vi "Config.vi"() -> ()   [LabVIEW 2020]
uses:
  Database/Global1.vi
  Global_Variable/Global.vi
  Global_Variable/A131258.vi
  <vilib>/Utility/config.llb/NI_LVConfig.lvlib
panel:
  in  "系数":bool
  in  "产品型号":string(combo)
  in  "删除":bool
  in  "确定":bool
  in  "添加":bool
  in  "退出":bool
  in  "更新":bool
  in  "选项卡控件":enum32{"产品参数", "系统参数"}(tab)
  in  "启用第二段监控":bool
  in  "判定框范围":string[][](table)=[["°"], ["N"], ["°"], ["N"], ["°"], ["N"], ["°"], ["N"]]
  in  "结果判定参数":string[][](table)=[["N"], ["N"], ["N"], ["N"], ["N"], ["N"], ["N"], ["N"], ["N"]]
  in  "工位滤波":cluster{"启用滤波":bool, "滤波系数":dbl}
  in  "系统参数设置":string[][](table)=[[""], [""], [""], [""]]
  # "上转向轴组件压装"
types:
  T1 = enum8{"Enabled", "Disabled", "Disabled and Grayed Out"}
  T2 = typedef "NI_LVConfig.lvlib/Config Data RefNum.ctl" = refnum<k1>
  T3 = cluster{"用户编号":string, "用户名":string, "用户密码(密文)":string, "用户权限":string}
  T4 = cluster{"[0]":cluster{string, dbl, dbl}, "[1]":cluster{string, dbl, dbl}, "[2]":cluster{string, dbl, dbl}, "[3]":cluster{string, dbl, dbl}}
  T5 = cluster{"[0]":cluster{string, dbl, dbl}, "[1]":cluster{string, dbl, dbl}, "[2]":cluster{string, dbl, dbl}, "[3]":cluster{string, dbl, dbl}, "[4]":cluster{string, dbl, dbl}}
  T6 = cluster{"[0]":cluster{string, dbl, dbl}, "[1]":cluster{string, dbl, dbl}, "[2]":cluster{string, dbl, dbl}}
  T7 = cluster{"第一段判定框位移":cluster{"单位":string, "下限":dbl, "上限":dbl}, "第一段判定框压力":cluster{"单位":string, "下限":dbl, "上限":dbl}, "低二段判定框位移":cluster{"单位":string, "下限":dbl, "上限":dbl}, "第二段判定框压力":cluster{"单位":string, "下限":dbl, "上限":dbl}}
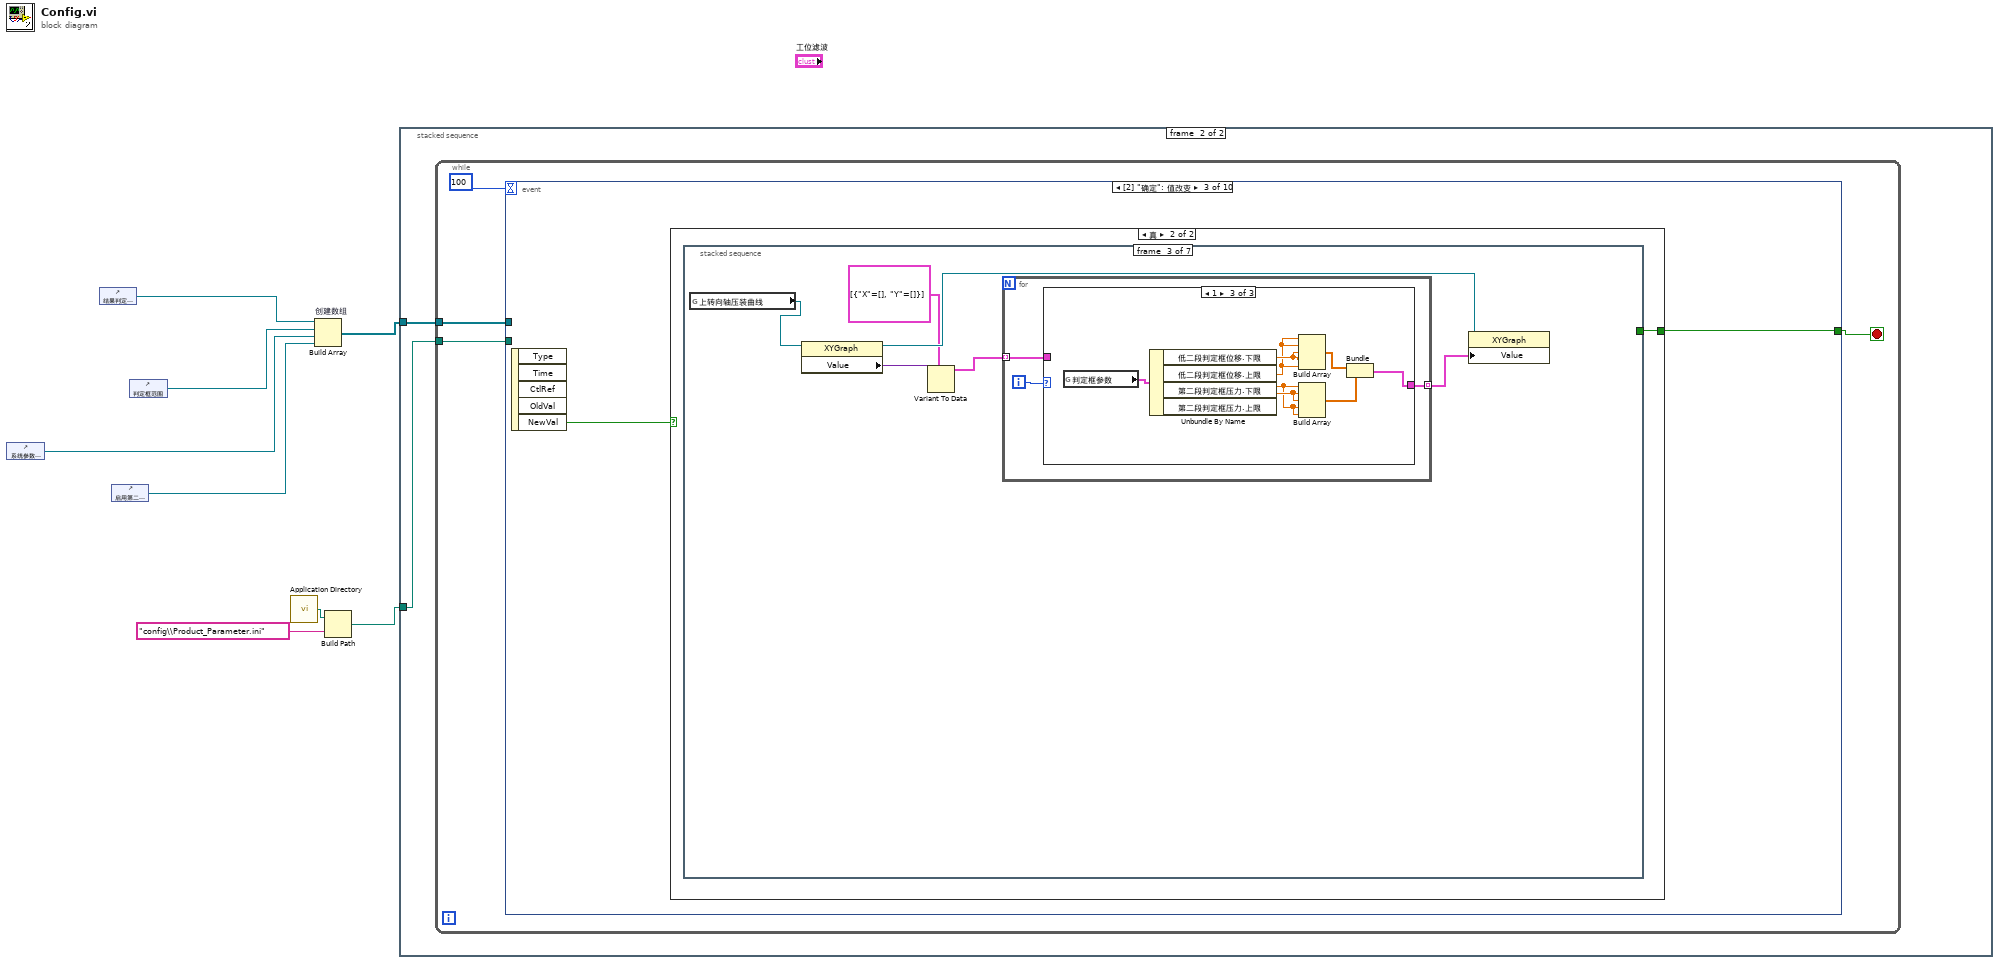
[diagram p0: block diagram]
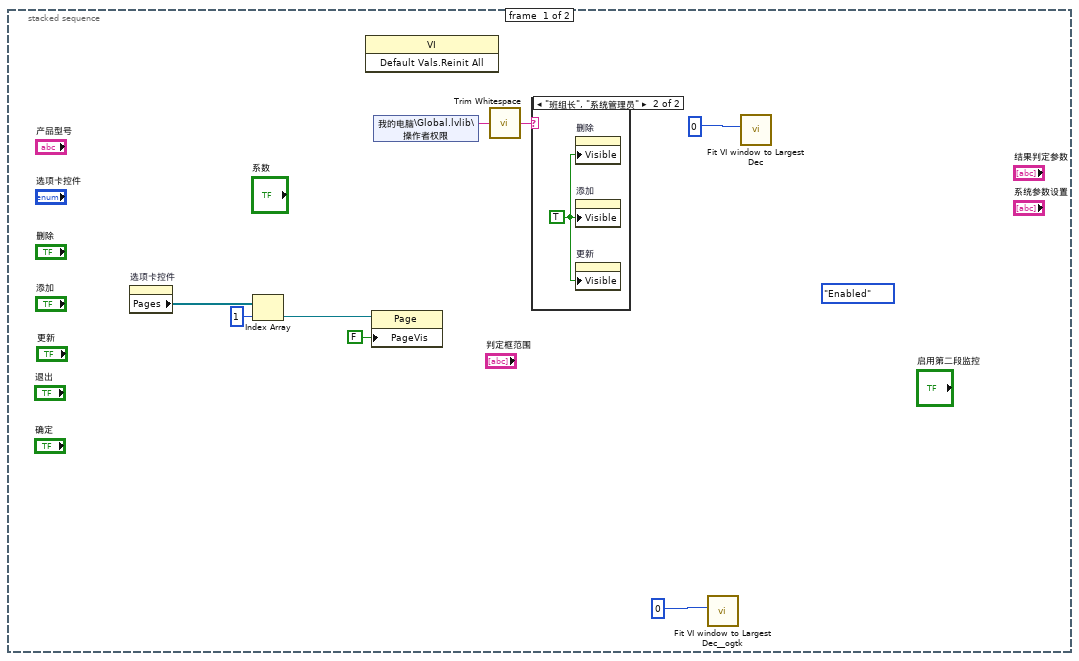
[diagram p2: hidden frame]
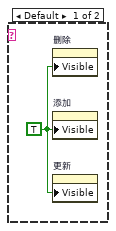
[diagram p3: hidden frame]
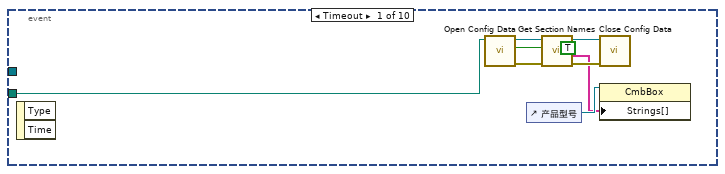
[diagram p4: hidden frame]
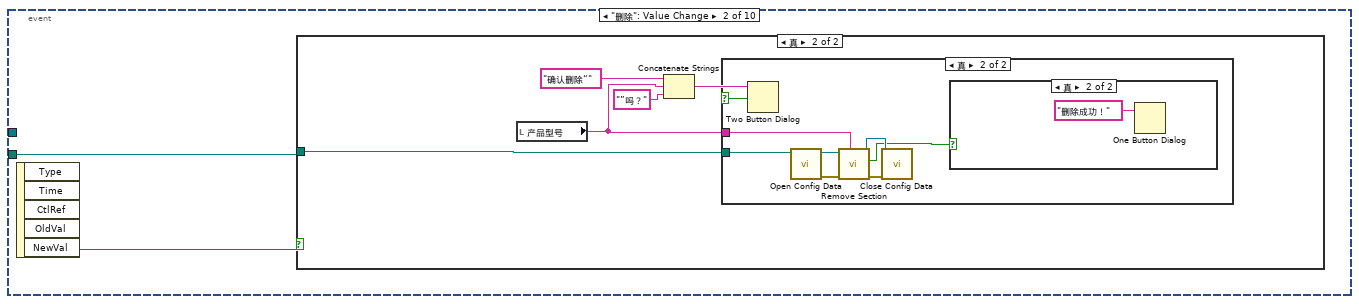
[diagram p5: hidden frame]
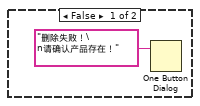
[diagram p8: hidden frame]
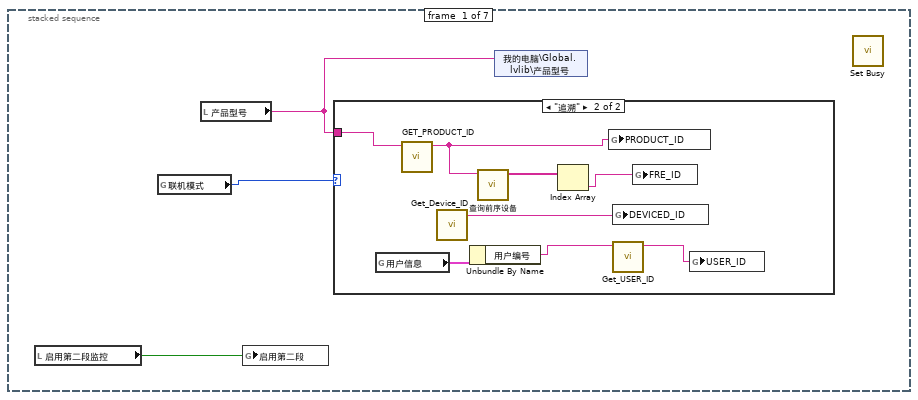
[diagram p10: hidden frame]
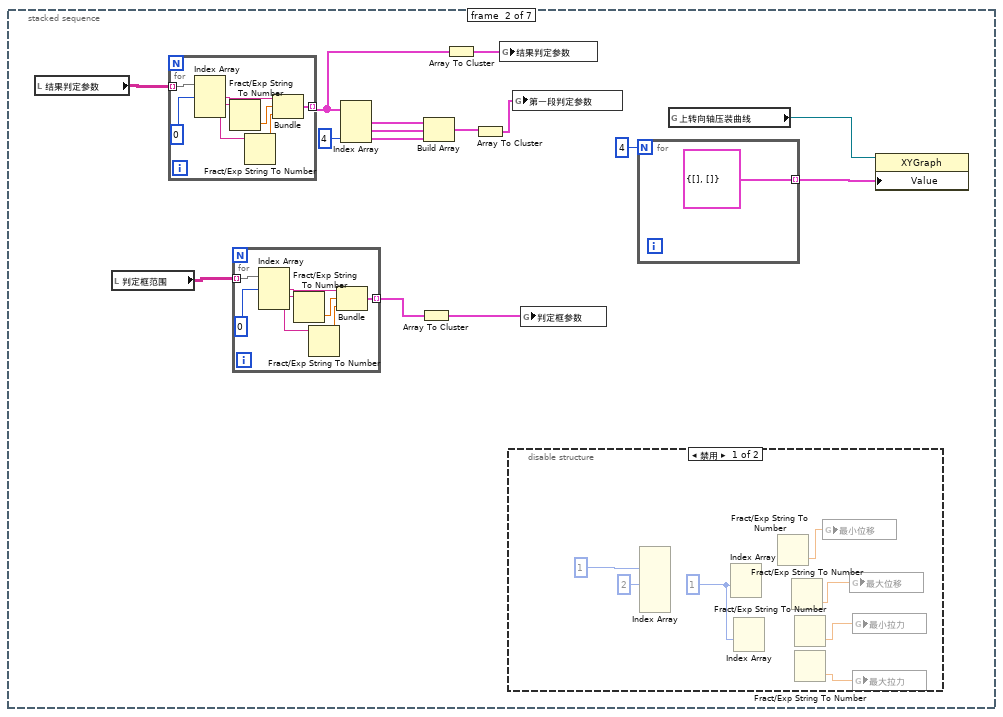
[diagram p12: hidden frame]
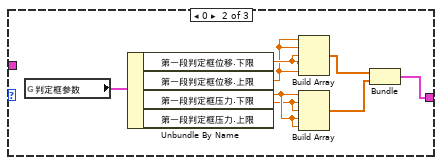
[diagram p15: hidden frame]
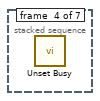
[diagram p16: hidden frame]
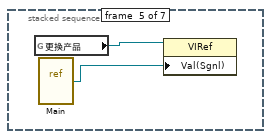
[diagram p17: hidden frame]
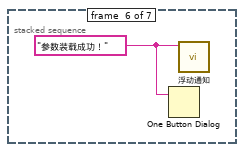
[diagram p18: hidden frame]
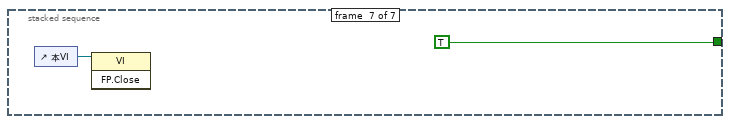
[diagram p19: hidden frame]
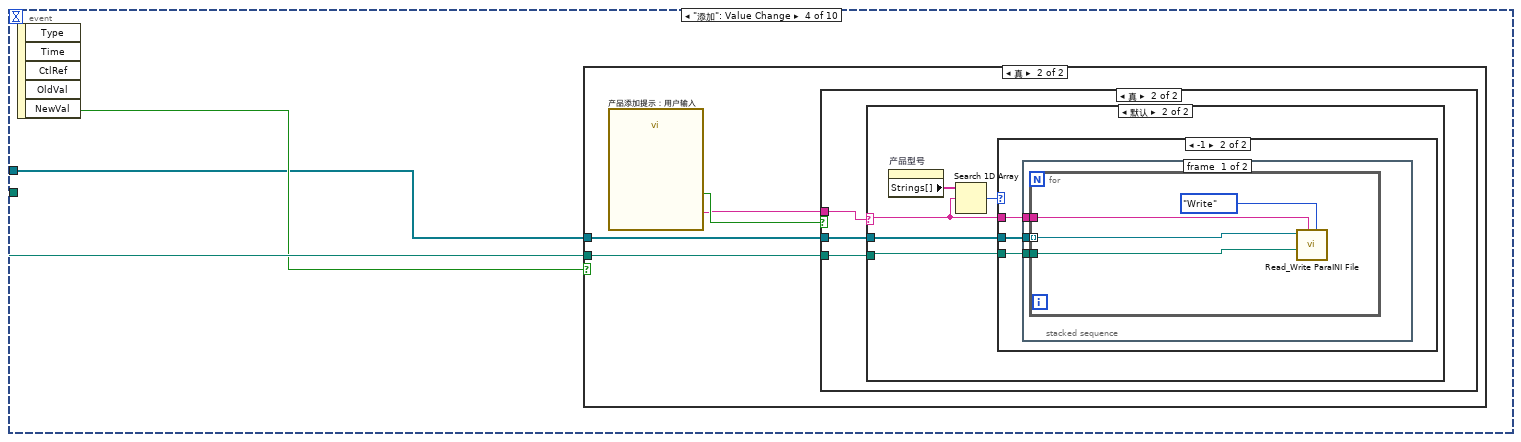
[diagram p20: hidden frame]
diagram:
  n1 = control-ref of="系统参数设置"() -> (w5:refnum<vi>)
  n2 = control-ref of="结果判定参数"() -> (w4:refnum<vi>)
  n3 = control-ref of="启用第二段监控"() -> (w1:refnum<vi>)
  n4 = control-ref of="判定框范围"() -> (w2:refnum<vi>)
  n5 = call <vilib>:"Application Directory.vi"() -> ("Application Directory"=w7:path)
  n6 = Build Array "创建数组"(w4, w2, w5, w1) -> (w8:refnum<vi>[])
  n7 = Build Path(base path=w7, name or relative path="config\\Product_Parameter.ini" ("名称或相对路径")) -> (appended path=w6:path)
  n8 = stacked-sequence {
    tunnel: w8 -> [_ w19]
    tunnel: w6 -> [_ w20]
    frame #0 {
      (unwired) T1."Enabled" ("禁用")
      n9 = property on="选项卡控件" class="TabCtl (严格)"() -> ("Pages"=w11:refnum<vi>[])  [unwired: 2 in, 2 out]
      n10 = Index Array(array=w11, index=1 ("索引")) -> (element=w12:refnum<vi>)
      n11 = invoke class="VI" method="Default Vals.Reinit All"() -> ()  [unwired: 3 in, 3 out]
      n12 = property class="Page"(reference=w12, "PageVis"=FALSE ("选项卡可见")) -> ()  [unwired: 1 in, 2 out]
      n13 = shared-variable "我的电脑\\Global.lvlib\\操作者权限"() -> (w16:string)  [unwired: 1 in, 1 out]
      n14 = call <vilib>:"Trim Whitespace.vi"("string"=w16) -> ("trimmed string"=w15:string)  [unwired: 1 in]
      n15 = case shown="\"班组长\", \"系统管理员\"" w15 {
        frame Default {
          w17 = TRUE ("可见")
          n16 = property on="删除" class="Bool (严格)"("Visible"=w17) -> ()  [unwired: 2 in, 2 out]
          n17 = property on="添加" class="Bool (严格)"("Visible"=w17) -> ()  [unwired: 2 in, 2 out]
          n18 = property on="更新" class="Bool (严格)"("Visible"=w17) -> ()  [unwired: 2 in, 2 out]
        }
        frame "班组长", "系统管理员" {
          w18 = TRUE ("可见")
          n19 = property on="删除" class="Bool (严格)"("Visible"=w18) -> ()  [unwired: 2 in, 2 out]
          n20 = property on="添加" class="Bool (严格)"("Visible"=w18) -> ()  [unwired: 2 in, 2 out]
          n21 = property on="更新" class="Bool (严格)"("Visible"=w18) -> ()  [unwired: 2 in, 2 out]
        }
      }
      n22 = call <userlib>:"Fit VI window to Largest Dec__ogtk.vi"("border spacing (2 px)"=0) -> ()  [unwired: 5 in, 2 out]
      n23 = call "Fit VI window to Largest Dec.vi"("border spacing (2 px)"=0) -> ()  [unwired: 5 in, 2 out]
    }
    frame #1 {
      n24 = while {
        tunnel: w20 -> [w24]
        tunnel: w19 -> [w21]
        stop <- w23 stop-if-true
        n25 = event shown="[2] \"确定\": 值改变" {
          selector: _ -> [_ _ _ _ _ _ _ _ _ _]
          dyn-events: _ -> [_ _ _ _ _ _ _ _ _ _]
          timeout: 100 -> [_ _ _ _ _ _ _ _ _ _]
          tunnel: w24 -> [w27 w34 _ w136 w164 _ w187 _ _ _]
          tunnel: [_ _ w50 _ _ TRUE _ _ _ TRUE] -> w23
          tunnel: w21 -> [_ _ _ w134 w162 _ w185 _ _ _]
          event Timeout {
            n26 = event-data() -> ()  [unwired: 1 in, 2 out]
            n27 = call <vilib>:"Open Config Data.vi"("create file if necessary (T)"=TRUE, "configuration file path"=w27) -> ("error out"=w29:errorcluster, "refnum"=w28:T2)  [unwired: 7 in, 1 out]
            n28 = control-ref of="产品型号"() -> (w26:refnum<vi>)
            n29 = call <vilib>:"Get Section Names.vi"("error in (no error)"=w29, "refnum"=w28) -> ("error out"=w31:errorcluster, "section names"=w25:string[], "refnum out"=w30:T2)  [unwired: 7 in]
            n30 = call <vilib>:"Close Config Data.vi"("error in (no error)"=w31, "refnum"=w30) -> ()  [unwired: 8 in, 2 out]
            n31 = property on="属性节点" class="CmbBox"(reference=w26, "Strings[]"=w25) -> ()  [unwired: 1 in, 2 out]
          }
          event "删除": Value Change {
            n32 = event-data() -> ("NewVal"=w33:bool)  [unwired: 1 in, 4 out]
            n33 = case shown="真" w33 {
              tunnel: w34 -> [_ w36]
              frame False {
              }
              frame True {
                n34 = local read "产品型号"() -> (w35:string)
                n35 = Concatenate Strings("确认删除“", w35, "”吗？") -> (w38:string)
                n36 = Two Button Dialog(message=w38) -> (T button?=w37:bool)  [unwired: 2 in]
                n37 = case shown="真" w37 {
                  tunnel: w36 -> [_ w42]
                  tunnel: w35 -> [_ w41]
                  frame False {
                  }
                  frame True {
                    n38 = call <vilib>:"Open Config Data.vi"("configuration file path"=w42) -> ("error out"=w44:errorcluster, "refnum"=w47:T2)  [unwired: 8 in, 1 out]
                    n39 = call <vilib>:"Remove Section.vi"("section"=w41, "error in (no error)"=w44, "refnum"=w47) -> ("error out"=w46:errorcluster, "section exists?"=w43:bool, "refnum out"=w45:T2)  [unwired: 6 in]
                    n40 = call <vilib>:"Close Config Data.vi"("error in (no error)"=w46, "refnum"=w45) -> ()  [unwired: 8 in, 2 out]
                    n41 = case shown="真" w43 {
                      frame False {
                        n42 = One Button Dialog(message="删除失败！\n请确认产品存在！" ("消息")) -> ()  [unwired: 1 in, 1 out]
                      }
                      frame True {
                        n43 = One Button Dialog(message="删除成功！" ("消息")) -> ()  [unwired: 1 in, 1 out]
                      }
                    }
                  }
                }
              }
            }
          }
          event "确定": Value Change {
            n44 = event-data() -> ("NewVal"=w51:bool)  [unwired: 1 in, 4 out]
            n45 = case shown="真" w51 {
              tunnel: [_ w52] -> w50
              frame False {
              }
              frame True {
                n46 = stacked-sequence {
                  tunnel: [_ _ _ _ _ _ TRUE] -> w52
                  frame #0 {
                    n47 = local read "启用第二段监控"() -> (w53:bool)
                    n48 = global read "Global1.vi" "联机模式"() -> (w55:enum16{"单机", "追溯"})
                    n49 = local read "产品型号"() -> (w54:string)
                    n50 = global write "Global.vi" "启用第二段"(w53) -> ()
                    n51 = case shown="\"追溯\"" w55 {
                      tunnel: w54 -> [_ w63]
                      frame "单机", Default {
                      }
                      frame "追溯" {
                        n52 = global read "Global1.vi" "用户信息"() -> (w61:T3)
                        n53 = call "GET_PRODUCT_ID.vi"("PRODFUCT_NAME"=w63) -> ("PRODUCT_ID"=w59:string)  [unwired: 10 in]
                        n54 = call "Get_Device_ID.vi"() -> ("Device_ID"=w57:string)  [unwired: 10 in, 1 out]
                        n55 = Unbundle By Name(w61) -> ("用户编号"=w60:string)
                        n56 = call "查询前序设备.vi"("PRODUCT_ID"=w59) -> ("前序工位"=w62:string[])  [unwired: 10 in]
                        n57 = Index Array(array=w62) -> (element=w58:string)  [unwired: 1 in]
                        n58 = global write "Global.vi" "PRODUCT_ID"(w59) -> ()
                        n59 = global write "Global.vi" "DEVICED_ID"(w57) -> ()
                        n60 = call "Get_USER_ID.vi"("USER_EMPLOYEE_ID"=w60) -> ("USER_ID"=w56:string)  [unwired: 9 in, 1 out]
                        n61 = global write "Global.vi" "FRE_ID"(w58) -> ()
                        n62 = global write "Global.vi" "USER_ID"(w56) -> ()
                      }
                    }
                    n63 = shared-variable "我的电脑\\Global.lvlib\\产品型号"(w54) -> ()  [unwired: 1 in, 1 out]
                    n64 = call <vilib>:"Set Busy.vi"() -> ()  [unwired: 10 in, 2 out]
                  }
                  frame #1 {
                    n65 = local read "结果判定参数"() -> (w78:string[][])
                    n66 = local read "判定框范围"() -> (w77:string[][])
                    n67 = for {
                      tunnel: w78 -> [w98] mode=indexing
                      tunnel: [w100] -> w68 mode=indexing
                      n68 = Index Array(array=w98, index #1=0) -> (element #1=w99:string, element #2=w97:string, element #3=w96:string)  [unwired: 2 in]
                      n69 = Fract/Exp String To Number(string=w97) -> (number=w102:dbl)  [unwired: 3 in, 1 out]
                      n70 = Fract/Exp String To Number(string=w96) -> (number=w101:dbl)  [unwired: 3 in, 1 out]
                      n71 = Bundle(w99, w102, w101) -> (w100:cluster{string, dbl, dbl})  [unwired: 1 in]
                    }
                    n72 = for {
                      tunnel: w77 -> [w90] mode=indexing
                      tunnel: [w92] -> w76 mode=indexing
                      n73 = Index Array(array=w90, index #1=0) -> (element #1=w91:string, element #2=w89:string, element #3=w88:string)  [unwired: 2 in]
                      n74 = Fract/Exp String To Number(string=w89) -> (number=w94:dbl)  [unwired: 3 in, 1 out]
                      n75 = Fract/Exp String To Number(string=w88) -> (number=w93:dbl)  [unwired: 3 in, 1 out]
                      n76 = Bundle(w91, w94, w93) -> (w92:cluster{string, dbl, dbl})  [unwired: 1 in]
                    }
                    n77 = Index Array(array=w68, index #3=4 ("索引")) -> (element #1=w71:cluster{string, dbl, dbl}, element #2=w70:cluster{string, dbl, dbl}, element #3=w69:cluster{string, dbl, dbl})  [unwired: 2 in]
                    n78 = Array To Cluster(array=w76) -> (cluster=w64:T4)
                    n79 = Build Array(w71, w70, w69) -> (w66:cluster{string, dbl, dbl}[])
                    n80 = Array To Cluster(array=w68) -> (cluster=w67:T5)
                    n81 = Array To Cluster(array=w66) -> (cluster=w65:T6)
                    n82 = global write "Global.vi" "结果判定参数"(w67) -> ()
                    n83 = disable-structure shown="禁用" {
                      frame Disabled {
                        w80 = 1 ("索引")
                        n84 = Index Array(index (row) #1=1 ("索引 (行)"), index (row) #2=2 ("索引 (行)")) -> ()  [unwired: 5 in, 3 out]
                        n85 = Index Array(index #1=w80) -> ()  [unwired: 2 in, 2 out]
                        n86 = Index Array(index #1=w80) -> ()  [unwired: 2 in, 2 out]
                        n87 = Fract/Exp String To Number() -> (number=w85:dbl)  [unwired: 4 in, 1 out]
                        n88 = Fract/Exp String To Number() -> (number=w84:dbl)  [unwired: 4 in, 1 out]
                        n89 = Fract/Exp String To Number() -> (number=w83:dbl)  [unwired: 4 in, 1 out]
                        n90 = Fract/Exp String To Number() -> (number=w82:dbl)  [unwired: 4 in, 1 out]
                        n91 = global write "判定参数.vi" "最小位移"(w85) -> ()
                        n92 = global write "判定参数.vi" "最大位移"(w84) -> ()
                        n93 = global write "判定参数.vi" "最小拉力"(w83) -> ()
                        n94 = global write "判定参数.vi" "最大拉力"(w82) -> ()
                      }
                      frame Enabled {
                      }
                    }
                    n95 = global write "Global.vi" "第一段判定参数"(w65) -> ()
                    n96 = global write "Global.vi" "判定框参数"(w64) -> ()
                    n97 = for {
                      N: 4 -> [_]
                      tunnel: [cluster{dbl[], dbl[]} {[], []}] -> w74 mode=indexing
                    }
                    n98 = global read "A131258.vi" "上转向轴压装曲线"() -> (w73:refnum<vi>)
                    n99 = property class="XYGraph"(reference=w73, "Value"=w74) -> ()  [unwired: 1 in, 2 out]
                  }
                  frame #2 {
                    n100 = global read "A131258.vi" "上转向轴压装曲线"() -> (w103:refnum<vi>)
                    n101 = property class="XYGraph"(reference=w103) -> (reference out=w108:refnum<vi>, "Value"=w106:variant)  [unwired: 1 in, 1 out]
                    n102 = Variant To Data(type=cluster{"X":dbl[], "Y":dbl[]}[] [{"X"=[], "Y"=[]}], Variant=w106) -> (data=w105:cluster{"X":dbl[], "Y":dbl[]}[])  [unwired: 1 in, 1 out]
                    n103 = for {
                      tunnel: [w110] -> w107 mode=indexing
                      tunnel: w105 -> [w109] mode=indexing
                      i -> [w111]
                      n104 = case shown="1" w111 {
                        tunnel: [w112 w113 w122] -> w110
                        tunnel: w109 -> [w112 _ _]
                        frame Default {
                        }
                        frame 0 {
                          n105 = global read "Global.vi" "判定框参数"() -> (w114:T7)
                          n106 = Unbundle By Name(w114) -> ("第一段判定框位移.下限"=w118:dbl, "第一段判定框位移.上限"=w117:dbl, "第一段判定框压力.下限"=w116:dbl, "第一段判定框压力.上限"=w115:dbl)
                          n107 = Build Array(w117, w117, w118, w118, w117) -> (w120:dbl[])
                          n108 = Build Array(w116, w115, w115, w116, w116) -> (w119:dbl[])
                          n109 = Bundle(w120, w119) -> (w113:cluster{dbl[], dbl[]})  [unwired: 1 in]
                        }
                        frame 1 {
                          n110 = global read "Global.vi" "判定框参数"() -> (w128:T7)
                          n111 = Unbundle By Name(w128) -> ("低二段判定框位移.下限"=w125:dbl, "低二段判定框位移.上限"=w121:dbl, "第二段判定框压力.下限"=w126:dbl, "第二段判定框压力.上限"=w127:dbl)
                          n112 = Build Array(w121, w121, w125, w125, w121) -> (w123:dbl[])
                          n113 = Build Array(w126, w127, w127, w126, w126) -> (w124:dbl[])
                          n114 = Bundle(w123, w124) -> (w122:cluster{dbl[], dbl[]})  [unwired: 1 in]
                        }
                      }
                    }
                    n115 = property class="XYGraph"(reference=w108, "Value"=w107) -> ()  [unwired: 1 in, 2 out]
                  }
                  frame #3 {
                    n116 = call <vilib>:"Unset Busy.vi"() -> ()  [unwired: 11 in, 1 out]
                  }
                  frame #4 {
                    n117 = global read "Global.vi" "更换产品"() -> (w130:refnum<vi>)
                    n118 = vi-ref "Main.vi"() -> (w129:refnum<vi>)
                    n119 = property class="VIRef"(reference=w130, "Val(Sgnl)"=w129) -> ()  [unwired: 1 in, 2 out]
                  }
                  frame #5 {
                    w131 = "参数装载成功！" ("消息")
                    n120 = One Button Dialog(message=w131) -> ()  [unwired: 1 in, 1 out]
                    n121 = call "浮动通知.vi"("通知内容"=w131) -> ()  [unwired: 11 in]
                  }
                  frame #6 {
                    n122 = control-ref of="本VI"() -> (w132:refnum<vi>)
                    n123 = invoke class="VI" method="FP.Close"(reference=w132) -> ()  [unwired: 2 in, 3 out]
                  }
                }
              }
            }
          }
          event "添加": Value Change {
            n124 = event-data() -> ("NewVal"=w135:bool)  [unwired: 1 in, 4 out]
            n125 = case shown="真" w135 {
              tunnel: w136 -> [_ w140]
              tunnel: w134 -> [_ w137]
              frame False {
              }
              frame True {
                n126 = call "产品添加提示：用户输入"() -> ("产品型号"=w138:string, "确定"=w139:bool)  [unwired: 17 in, 1 out]
                n127 = case shown="真" w139 {
                  tunnel: w140 -> [_ w143]
                  tunnel: w138 -> [_ w142]
                  tunnel: w137 -> [_ w141]
                  frame False {
                  }
                  frame True {
                    n128 = case shown="默认" w142 {
                      selector: w142 -> [_ w147]
                      tunnel: w143 -> [_ w149]
                      tunnel: w141 -> [_ w145]
                      frame "" {
                        n129 = One Button Dialog(message="产品名称不得为空!" ("text")) -> ()  [unwired: 1 in, 1 out]
                      }
                      frame Default {
                        n130 = property on="产品型号" class="CmbBox"() -> ("Strings[]"=w148:string[])  [unwired: 2 in, 2 out]
                        n131 = Search 1D Array(1D array=w148, element=w147) -> (index of element=w146:i32)  [unwired: 1 in]
                        n132 = case shown="-1" w146 {
                          tunnel: w149 -> [_ w153]
                          tunnel: w147 -> [_ w152]
                          tunnel: w145 -> [_ w151]
                          frame Default {
                            n133 = One Button Dialog(message="产品已存在！" ("消息")) -> ()  [unwired: 1 in, 1 out]
                          }
                          frame -1 {
                            n134 = stacked-sequence {
                              tunnel: w153 -> [w156 _]
                              tunnel: w152 -> [w155 _]
                              tunnel: w151 -> [w154 _]
                              frame #0 {
                                n135 = for {
                                tunnel: w156 -> [w160]
                                tunnel: w155 -> [w157]
                                tunnel: w154 -> [w159] mode=indexing
                                n136 = call "Read_Write ParaINI File.vi"("Mode"=enum16{"Read", "Write"}."Write", "Section"=w157, "Filepath"=w160, "Ctl Refnum"=w159) -> ()  [unwired: 7 in, 1 out]
                                }
                              }
                              frame #1 {
                                n137 = One Button Dialog(message="添加成功！" ("消息")) -> ()  [unwired: 1 in, 1 out]
                              }
                            }
                          }
                        }
                      }
                    }
                  }
                }
              }
            }
          }
          event "产品型号": Value Change {
            n138 = event-data() -> ("NewVal"=w163:string)  [unwired: 1 in, 4 out]
            n139 = stacked-sequence {
              tunnel: w164 -> [_ _ w168]
              tunnel: w163 -> [_ w166 _]
              tunnel: w162 -> [_ _ w167]
              frame #0 {
                n140 = control-ref of="本VI"() -> (w165:refnum<vi>)
                n141 = invoke class="VI" method="Default Vals.Reinit All"(reference=w165) -> ()  [unwired: 2 in, 3 out]
              }
              frame #1 {
                n142 = local write "产品型号"(w166) -> ()
              }
              frame #2 {
                n143 = disable-structure shown="启用" {
                  disable-tunnel: w168 -> [w169 w177]
                  disable-tunnel: w167 -> [_ w178]
                  frame Disabled {
                    n144 = for {
                      tunnel: [w173] -> w170 mode=indexing
                      tunnel: w169 -> [w172]
                      n145 = local read "产品型号"() -> (w171:string)
                      n146 = call "Read_Write ParaINI File.vi"("Mode"=enum16{"Read", "Write"}."Read", "Section"=w171, "Filepath"=w172, "Ctl Refnum"=w173) -> ()  [unwired: 7 in, 1 out]
                    }
                  }
                  frame Enabled {
                    n147 = local read "产品型号"() -> (w179:string)
                    n148 = call <vilib>:"Set Busy.vi"() -> ("error out"=w176:errorcluster)  [unwired: 10 in, 1 out]
                    n149 = call "Read_Write INI File.vi"("Mode"=enum16{"Read", "Write"}."Read", "Section"=w179, "error in"=w176, "Filepath"=w177, "Ctl Refnum"=w178) -> ("error out"=w175:errorcluster)  [unwired: 6 in]
                    n150 = call <vilib>:"Unset Busy.vi"("error in (no error)"=w175) -> ()  [unwired: 10 in, 1 out]
                  }
                }
              }
            }
          }
          event "退出": Value Change {
            n151 = event-data() -> ()  [unwired: 1 in, 5 out]
            n152 = control-ref of="本VI"() -> (w183:refnum<vi>)
            n153 = invoke class="VI" method="FP.Close"(reference=w183) -> (reference out=w181:refnum<vi>, error out=w182:errorcluster)  [unwired: 2 in, 1 out]
            n154 = Close Reference(reference=w181, error in (no error)=w182) -> ()  [unwired: 1 out]
          }
          event "更新": Value Change {
            n155 = event-data() -> ("NewVal"=w186:bool)  [unwired: 1 in, 4 out]
            n156 = case shown="真" w186 {
              tunnel: w187 -> [_ w190]
              tunnel: w185 -> [_ w188]
              frame False {
              }
              frame True {
                n157 = for {
                  tunnel: w190 -> [w197]
                  tunnel: [w196] -> w189
                  tunnel: w188 -> [w195] mode=indexing
                  n158 = local read "产品型号"() -> (w199:string)
                  n159 = call "Read_Write ParaINI File.vi"("Mode"=enum16{"Read", "Write"}."Write", "Section"=w199, "Filepath"=w197, "Ctl Refnum"=w195) -> ("error out"=w196:errorcluster)  [unwired: 7 in]
                }
                n160 = case shown="无错误" w189 {
                  frame No Error {
                    n161 = Wait (ms)(milliseconds to wait=u32 500 ("等待时间（毫秒）")) -> ()  [unwired: 1 out]
                    n162 = One Button Dialog(message="更新成功！" ("通知内容")) -> ()  [unwired: 1 in, 1 out]
                  }
                  frame Error {
                    n163 = Wait (ms)(milliseconds to wait=u32 500 ("等待时间（毫秒）")) -> ()  [unwired: 1 out]
                    n164 = call "浮动通知.vi"("通知内容"="更新失败！") -> ()  [unwired: 11 in]
                  }
                }
              }
            }
          }
          event "系数": Mouse Enter {
            n165 = event-data() -> ()  [unwired: 1 in, 4 out]
            n166 = property on="系数" class="Bool"("Colors [4]"=cluster{u32, u32}[] [{16777216, 16777216}] ("颜色[4]")) -> ()  [unwired: 2 in, 2 out]
          }
          event "系数": Value Change {
            n167 = event-data() -> ("NewVal"=w202:bool)  [unwired: 1 in, 5 out]
            n168 = property on="选项卡控件" class="TabCtl (严格)"() -> ("Pages"=w204:refnum<vi>[])  [unwired: 2 in, 2 out]
            n169 = Index Array(array=w204, index=1 ("索引")) -> (element=w203:refnum<vi>)
            n170 = property class="Page"(reference=w203, "PageVis"=w202) -> ()  [unwired: 1 in, 2 out]
          }
          event Panel Close {
            n171 = event-data() -> ()  [unwired: 1 in, 3 out]
          }
        }
      }
    }
  }
